vi "Latch Position.vi"(10 "Position":fxp<+/-,64,32>, 11 "Sensor":bool) -> (3 "Latched position":fxp<+/-,64,32>)   [LabVIEW 2013]
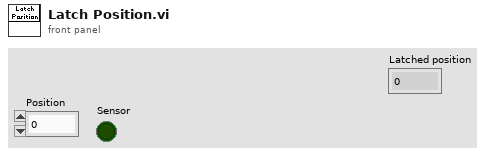
[diagram p1: front panel]
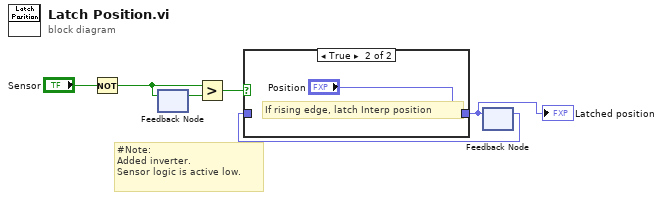
[diagram p0: block diagram]
diagram:
  # "#Note:\nAdded inverter.\nSensor logic is active low."
  n1 = Not(x="Sensor") -> (.not. x?=w1:bool)
  n2 = feedback-in #1(w1) -> ()
  n3 = feedback #1() -> (w6:bool)  [unwired: 1 in]
  n4 = Greater?(x=w1, y=w6) -> (0:w5:bool)
  n5 = feedback #2() -> (w4:fxp<+/-,64,32>)  [unwired: 1 in]
  n6 = case shown="True" w5 {
    tunnel: [w7 "Position"] -> w3
    tunnel: w4 -> [w7 _]
    frame False {
    }
    frame True {
      # "If rising edge, latch Interp position"
    }
  }
  "Latched position" <- w3
  n7 = feedback-in #2(w3) -> ()
